vi "Teleop.vi"(0 "Call Context":T10) -> (6 "SubState 3":T2, 8 "SubState 4":T2, 9 "SubState 5":T9, 10 "Loop 4 Data":T1, 11 "Loop 3 Data":T5, 14 "SubState 0":T2=enum."driver control", 15 "Loop 1 Data":T7, 16 "Loop 0 Data":T8, 17 "SubState 1":T2, 18 "Loop 2 Data":T6, 19 "SubState 2":T2)   [LabVIEW 2013]
uses:
  typedefs/state machine/subStates.ctl
  <vilib>/Rock Robotics/WPI/DriverStation/WPI_DriverStationDerivedRobotMode.ctl
  typedefs/state machine/singleUseSubstate.ctl
  typedefs/loop datatypes/Loop 0 Datatype.ctl
  typedefs/loop datatypes/Loop 1 Datatype.ctl
  typedefs/loop datatypes/Loop 2 Datatype.ctl
  typedefs/loop datatypes/Loop 3 Datatype.ctl
  <vilib>/Rock Robotics/WPI/Joystick/WPI_JoystickDevRef.ctl
  <vilib>/Rock Robotics/WPI/Joystick/WPI_JoystickDeviceEnum.ctl
  typedefs/loop datatypes/Loop 4 Datatype.ctl
  typedefs/fg_getset.ctl
  typedefs/vision/vision enable.ctl
  <vilib>/Rock Robotics/WPI/Joystick/WPI_JoystickGetSetRefNum.vi
panel:
  out "Drive to DC":bool
  out "JS3":T3
  out "JS1":T3
  out "JS2":T3
  out "Exit Value":i32=-1
  # "Teleoperated Loop Data and Substates"
  # "Drive Loop"
  # "Loop 1"
  # "Loop 2"
  # "Loop 3"
  # "Loop 4"
  # "Pneumatics Loop"
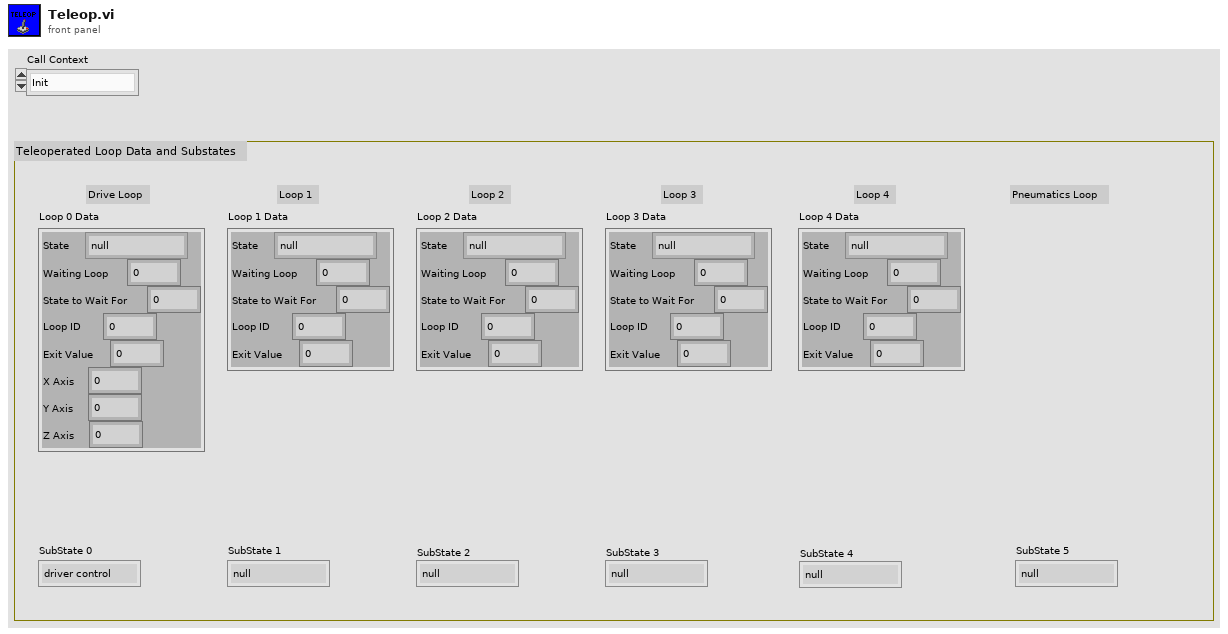
[diagram p1: front panel]
types:
  T1 = typedef "Loop 4 Datatype.ctl" = cluster{"State":T2, "Waiting Loop":i32, "State to Wait For":i32, "Loop ID":i32, "Exit Value":i32}
  T2 = typedef "subStates.ctl" = enum16{"null", "wait", "driver control", "auto", "manual override", "hold position", "rotate", "test", "end"}
  T3 = typedef "WPI_JoystickDevRef.ctl" = cluster{"Device":T4}
  T4 = typedef "WPI_JoystickDeviceEnum.ctl" = enum16{"USB 1", "USB 2", "USB 3", "USB 4", "Kinect 1", "Kinect 2"}
  T5 = typedef "Loop 3 Datatype.ctl" = cluster{"State":T2, "Waiting Loop":i32, "State to Wait For":i32, "Loop ID":i32, "Exit Value":i32}
  T6 = typedef "Loop 2 Datatype.ctl" = cluster{"State":T2, "Waiting Loop":i32, "State to Wait For":i32, "Loop ID":i32, "Exit Value":i32}
  T7 = typedef "Loop 1 Datatype.ctl" = cluster{"State":T2, "Waiting Loop":i32, "State to Wait For":i32, "Loop ID":i32, "Exit Value":i32}
  T8 = typedef "Loop 0 Datatype.ctl" = cluster{"State":T2, "Waiting Loop":i32, "State to Wait For":i32, "Loop ID":i32, "Exit Value":i32, "X Axis":dbl, "Y Axis":dbl, "Z Axis":dbl}
  T9 = typedef "singleUseSubstate.ctl" = enum16{"null", "wait", "shift high", "shift low", "end"}
  T10 = typedef "WPI_DriverStationDerivedRobotMode.ctl" = enum16{"Init", "Execute", "Stop"}
  T11 = cluster{"axis 1 (x)":dbl, "axis 2 (y)":dbl, "axis 3 (throttle)":dbl, "axis 4":dbl, "axis 5":dbl, "axis 6":dbl}
  T12 = typedef "vision enable.ctl" = enum16{"Enable", "Disable", "Stop"}
  T13 = typedef "fg_getset.ctl" = enum16{"Get", "Set"}
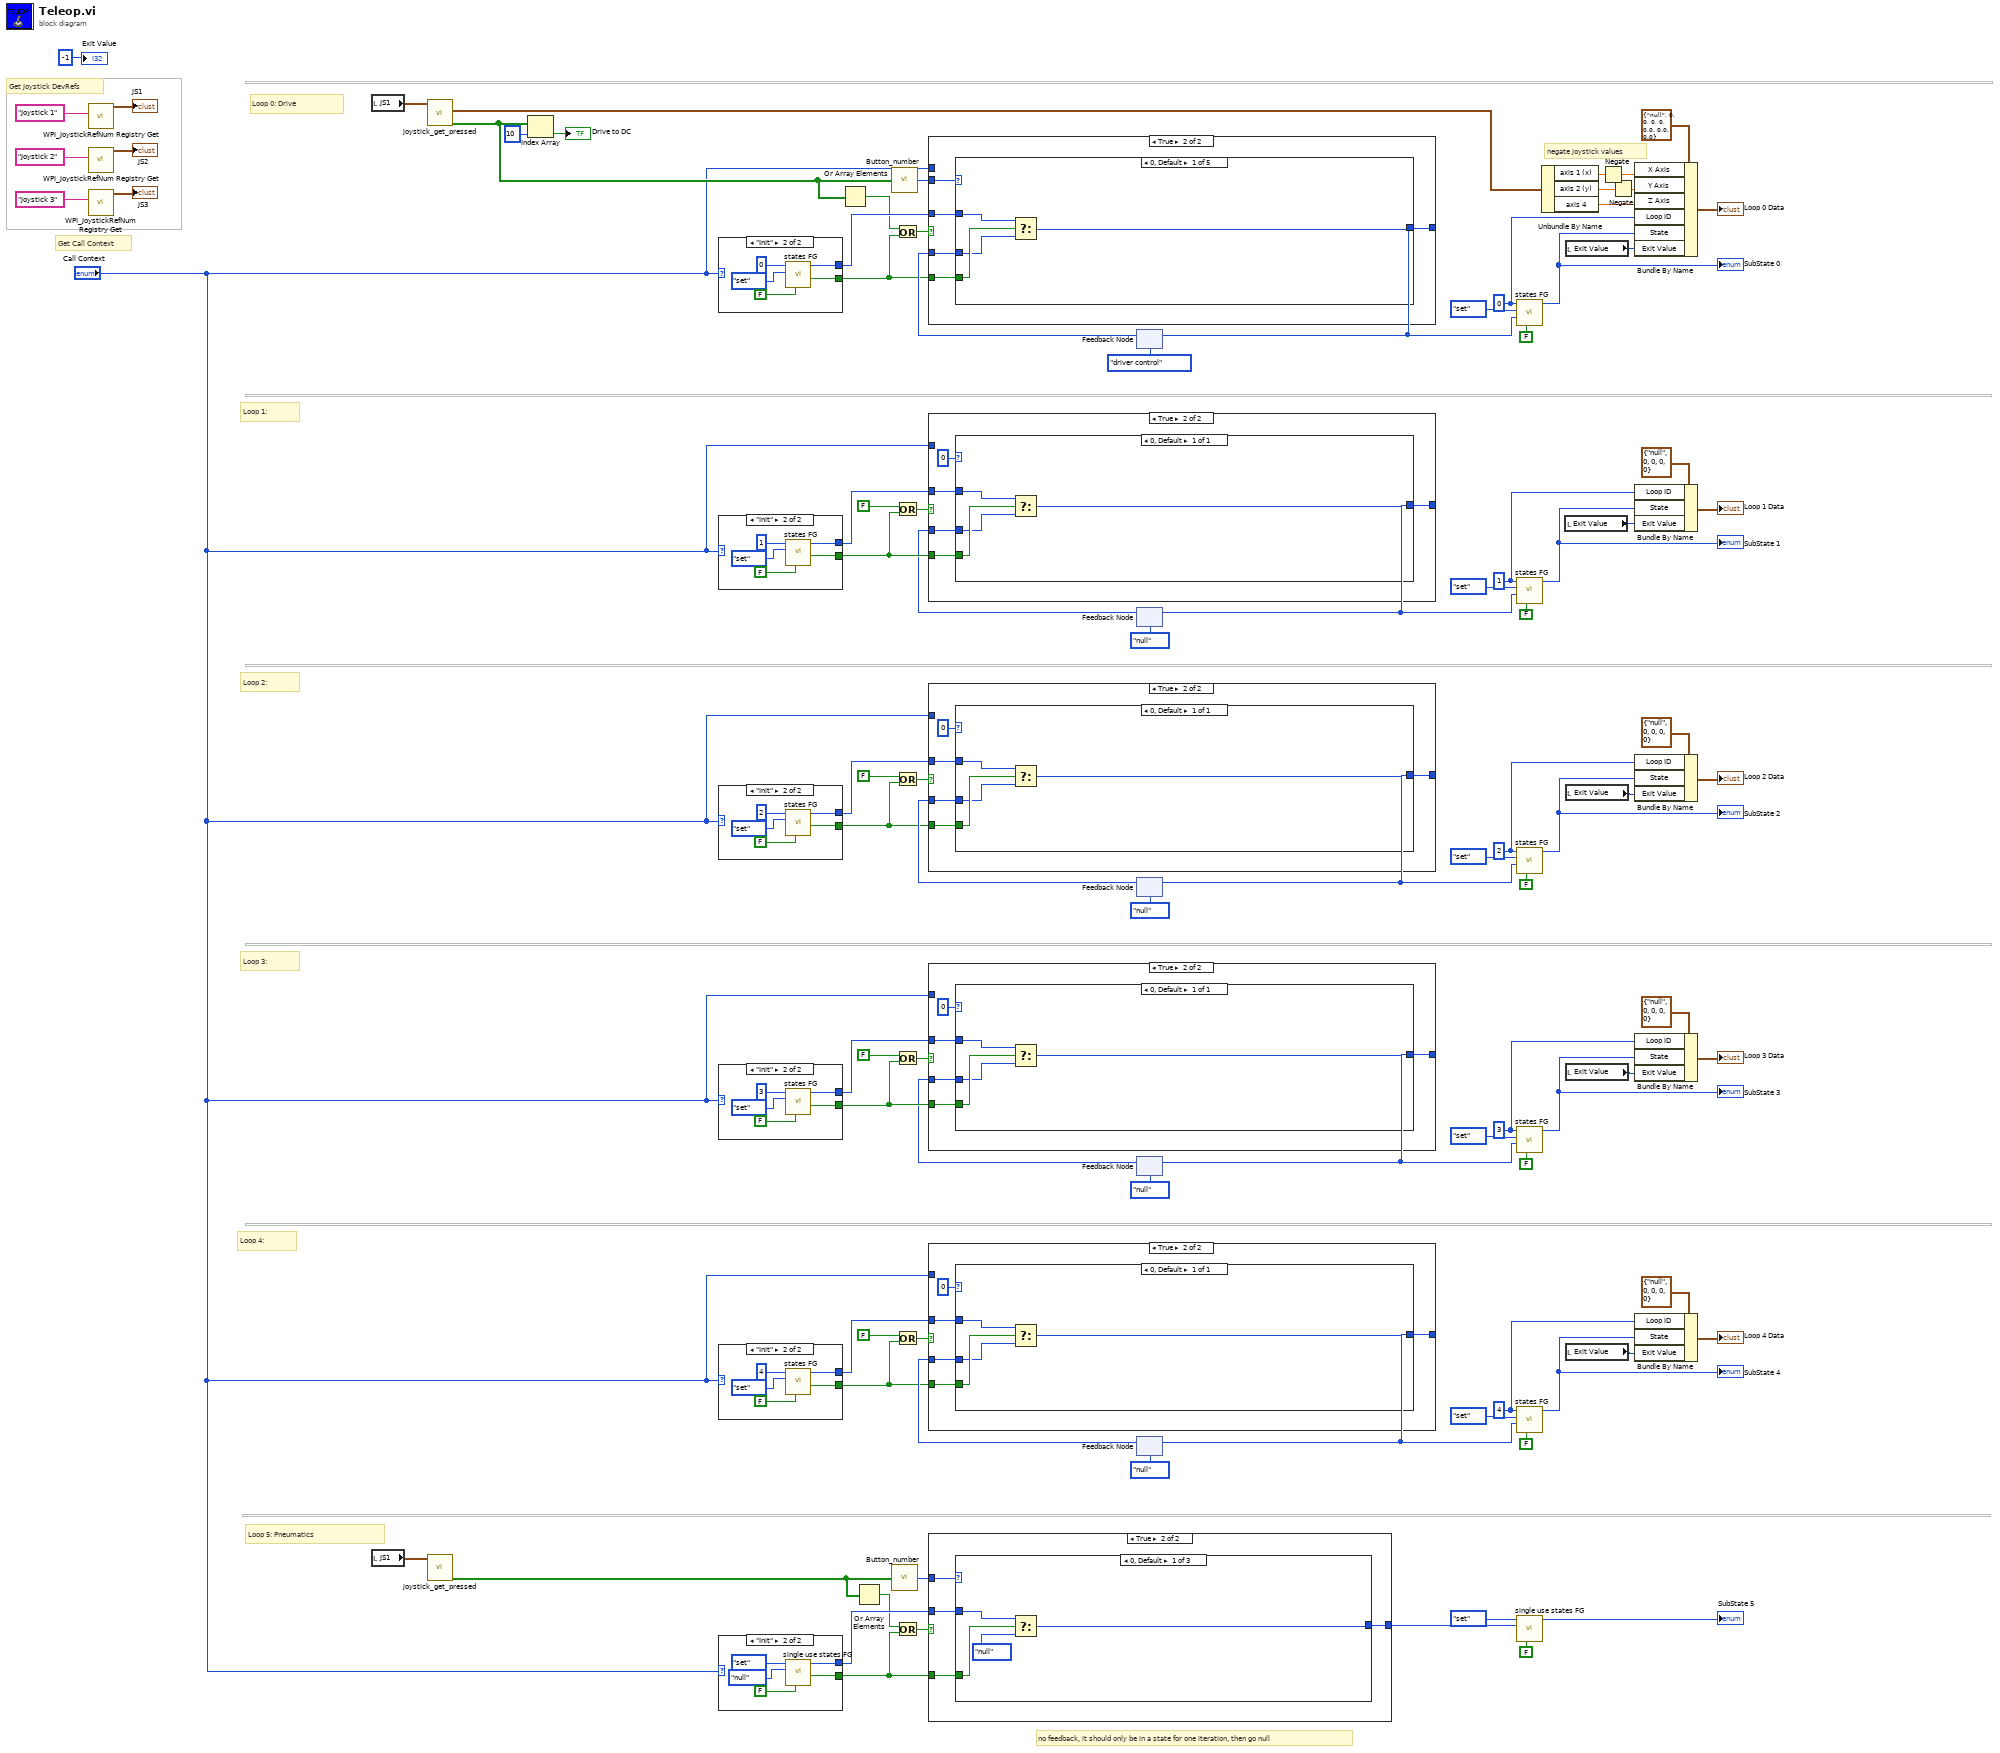
[diagram p0: block diagram]
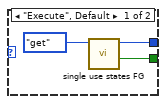
[diagram p2: hidden frame]
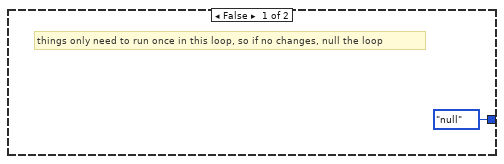
[diagram p3: hidden frame]
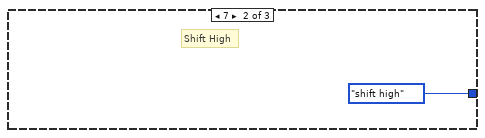
[diagram p4: hidden frame]
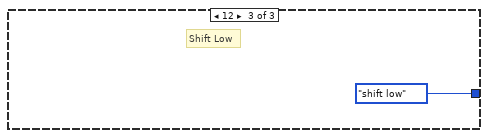
[diagram p5: hidden frame]
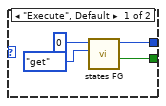
[diagram p6: hidden frame]
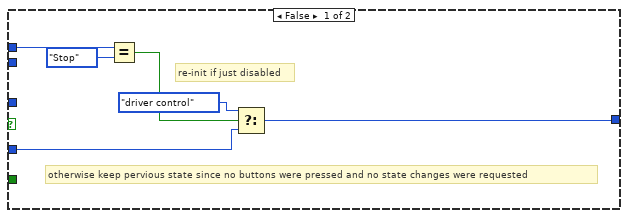
[diagram p7: hidden frame]
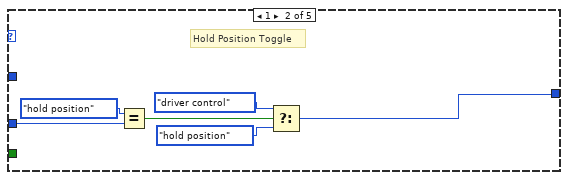
[diagram p8: hidden frame]
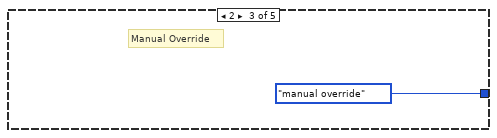
[diagram p9: hidden frame]
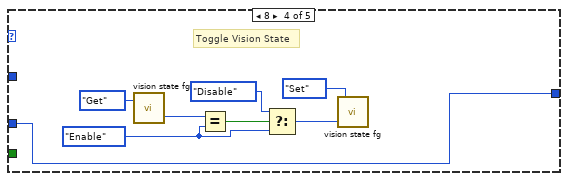
[diagram p10: hidden frame]
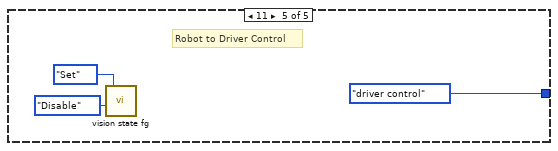
[diagram p11: hidden frame]
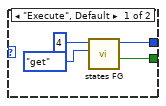
[diagram p12: hidden frame]
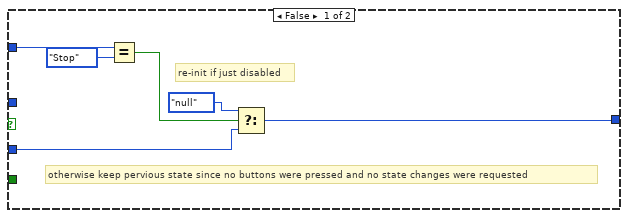
[diagram p13: hidden frame]
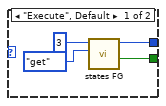
[diagram p14: hidden frame]
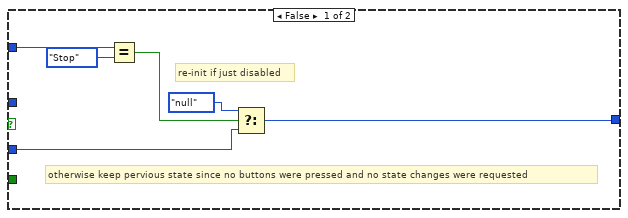
[diagram p15: hidden frame]
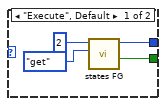
[diagram p16: hidden frame]
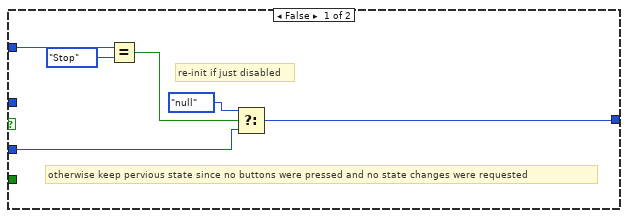
[diagram p17: hidden frame]
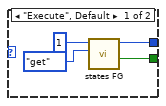
[diagram p18: hidden frame]
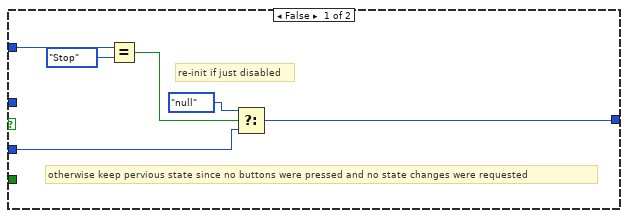
[diagram p19: hidden frame]
diagram:
  w39 = 0 ("Loop ID")
  w50 = 4 ("Loop ID")
  w65 = 3 ("Loop ID")
  w76 = 2 ("Loop ID")
  w94 = 1 ("Loop ID")
  # "no feedback, it should only be in a state for one iteration, then go null"
  # "negate joystick values"
  # "Loop 3:"
  # "Loop 2:"
  # "Loop 4:"
  # "Get Call Context"
  # "Get Joystick DevRefs"
  # "Loop 5: Pneumatics"
  # "Loop 1:"
  # "Loop 0: Drive"
  n1 = call <vilib>:"WPI_JoystickRefNum Registry Get.vi"("refnum name"="Joystick 1") -> ("JoystickDevRef"=→"JS1":T3)  [unwired: 9 in, 1 out]
  n2 = call <vilib>:"WPI_JoystickRefNum Registry Get.vi"("refnum name"="Joystick 2") -> ("JoystickDevRef"=→"JS2":T3)  [unwired: 9 in, 1 out]
  n3 = call <vilib>:"WPI_JoystickRefNum Registry Get.vi"("refnum name"="Joystick 3") -> ("JoystickDevRef"=→"JS3":T3)  [unwired: 9 in, 1 out]
  n4 = local read "JS1"() -> (w30:T3)
  n5 = local read "JS1"() -> (w12:T3)
  n6 = call "joystick_get_pressed.vi"("JoystickDevRef"=w30) -> ("Buttons Pressed?"=w20:bool[], "Axes"=w27:T11)  [unwired: 3 in, 2 out]
  n7 = call "joystick_get_pressed.vi"("JoystickDevRef"=w12) -> ("Buttons Pressed?"=w10:bool[])  [unwired: 3 in, 3 out]
  n8 = Index Array(array=w20, index=10) -> (element=→"Drive to DC":bool)
  n9 = case shown="\"Init\"" "Call Context" {
    tunnel: [w102 w107] -> w34
    tunnel: [w101 w105] -> w38
    frame "Execute", Default {
      n10 = call "states FG.vi"("menu (get)"=enum16{"set", "get"}."get", "Loop ID"=0) -> ("exit out"=w102:bool, "subState out"=w101:T2)  [unwired: 6 in, 2 out]
    }
    frame "Init" {
      n11 = call "states FG.vi"("exit in"=FALSE, "menu (get)"=enum16{"set", "get"}."set", "Loop ID"=0) -> ("exit out"=w107:bool, "subState out"=w105:T2)  [unwired: 5 in, 2 out]
    }
  }
  n12 = case shown="\"Init\"" "Call Context" {
    tunnel: [w111 w116] -> w100
    tunnel: [w110 w114] -> w96
    frame "Execute", Default {
      n13 = call "states FG.vi"("menu (get)"=enum16{"set", "get"}."get", "Loop ID"=1) -> ("exit out"=w111:bool, "subState out"=w110:T2)  [unwired: 6 in, 2 out]
    }
    frame "Init" {
      n14 = call "states FG.vi"("exit in"=FALSE, "menu (get)"=enum16{"set", "get"}."set", "Loop ID"=1) -> ("exit out"=w116:bool, "subState out"=w114:T2)  [unwired: 5 in, 2 out]
    }
  }
  n15 = case shown="\"Init\"" "Call Context" {
    tunnel: [w120 w125] -> w71
    tunnel: [w119 w123] -> w75
    frame "Execute", Default {
      n16 = call "states FG.vi"("menu (get)"=enum16{"set", "get"}."get", "Loop ID"=2) -> ("exit out"=w120:bool, "subState out"=w119:T2)  [unwired: 6 in, 2 out]
    }
    frame "Init" {
      n17 = call "states FG.vi"("exit in"=FALSE, "menu (get)"=enum16{"set", "get"}."set", "Loop ID"=2) -> ("exit out"=w125:bool, "subState out"=w123:T2)  [unwired: 5 in, 2 out]
    }
  }
  n18 = case shown="\"Init\"" "Call Context" {
    tunnel: [w129 w134] -> w70
    tunnel: [w128 w132] -> w66
    frame "Execute", Default {
      n19 = call "states FG.vi"("menu (get)"=enum16{"set", "get"}."get", "Loop ID"=3) -> ("exit out"=w129:bool, "subState out"=w128:T2)  [unwired: 6 in, 2 out]
    }
    frame "Init" {
      n20 = call "states FG.vi"("exit in"=FALSE, "menu (get)"=enum16{"set", "get"}."set", "Loop ID"=3) -> ("exit out"=w134:bool, "subState out"=w132:T2)  [unwired: 5 in, 2 out]
    }
  }
  n21 = case shown="\"Init\"" "Call Context" {
    tunnel: [w138 w143] -> w45
    tunnel: [w137 w141] -> w49
    frame "Execute", Default {
      n22 = call "states FG.vi"("menu (get)"=enum16{"set", "get"}."get", "Loop ID"=4) -> ("exit out"=w138:bool, "subState out"=w137:T2)  [unwired: 6 in, 2 out]
    }
    frame "Init" {
      n23 = call "states FG.vi"("exit in"=FALSE, "menu (get)"=enum16{"set", "get"}."set", "Loop ID"=4) -> ("exit out"=w143:bool, "subState out"=w141:T2)  [unwired: 5 in, 2 out]
    }
  }
  n24 = case shown="\"Init\"" "Call Context" {
    tunnel: [w148 w152] -> w16
    tunnel: [w147 w153] -> w15
    frame "Execute", Default {
      n25 = call "single use states FG.vi"("menu (get)"=enum16{"set", "get"}."get") -> ("exit out"=w148:bool, "substate out"=w147:T9)  [unwired: 7 in, 2 out]
    }
    frame "Init" {
      n26 = call "single use states FG.vi"("exit in"=FALSE, "substate"=singleUseSubstate."null", "menu (get)"=enum16{"set", "get"}."set") -> ("exit out"=w152:bool, "substate out"=w153:T9)  [unwired: 5 in, 2 out]
    }
  }
  n27 = Or Array Elements(Boolean array=w20) -> (logical OR=w19:bool)
  n28 = Or Array Elements(Boolean array=w10) -> (logical OR=w11:bool)
  n29 = call "Button_number.vi"("Button Array"=w20) -> ("Button Pressed"=w21:i32)
  n30 = call "Button_number.vi"("Button Array"=w10) -> ("Button Pressed"=w9:i32)
  n31 = Or(x=w19, y=w34) -> (x .or. y?=w42:bool)
  n32 = Or(x=FALSE, y=w100) -> (x .or. y?=w83:bool)
  n33 = Or(x=FALSE, y=w71) -> (x .or. y?=w79:bool)
  n34 = Or(x=FALSE, y=w70) -> (x .or. y?=w62:bool)
  n35 = Or(x=FALSE, y=w45) -> (x .or. y?=w53:bool)
  n36 = Or(x=w11, y=w16) -> (x .or. y?=w14:bool)
  n37 = case shown="True" w14 {
    tunnel: [singleUseSubstate."null" ("substate out") w157] -> w8
    tunnel: w15 -> [_ w158]
    tunnel: w16 -> [_ w156]
    tunnel: w9 -> [_ w155]
    frame False {
      # "things only need to run once in this loop, so if no changes, null the loop"
    }
    frame True {
      n38 = case shown="0, Default" w155 {
        tunnel: w158 -> [w161 _ _]
        tunnel: [w160 singleUseSubstate."shift high" ("f") singleUseSubstate."shift low" ("f")] -> w157
        tunnel: w156 -> [w162 _ _]
        frame 0, Default {
          n39 = Select(t=w161, s=w162, f=singleUseSubstate."null") -> (s? t:f=w160:T9)
        }
        frame 7 {
          # "Shift High"
        }
        frame 12 {
          # "Shift Low"
        }
      }
    }
  }
  n40 = feedback #1(subStates."driver control" ("Drive SubState")) -> (w41:T2)
  n41 = case shown="True" w42 {
    tunnel: w41 -> [w167 w174]
    tunnel: [w165 w173] -> w33
    tunnel: w38 -> [_ w175]
    tunnel: w34 -> [_ w172]
    tunnel: "Call Context" -> [w170 _]
    tunnel: w21 -> [_ w171]
    frame False {
      # "re-init if just disabled"
      # "otherwise keep pervious state since no buttons were pressed and no state changes were requested"
      n42 = Equal?(x=w170, y=WPI_DriverStationDerivedRobotMode."Stop") -> (x = y?=w168:bool)
      n43 = Select(t=subStates."driver control", s=w168, f=w167) -> (s? t:f=w165:T2)
    }
    frame True {
      n44 = case shown="0, Default" w171 {
        tunnel: w175 -> [w178 _ _ _ _]
        tunnel: w174 -> [w177 w185 _ w187 _]
        tunnel: [w176 w180 subStates."manual override" ("Drive SubState") w187 subStates."driver control" ("Drive SubState")] -> w173
        tunnel: w172 -> [w179 _ _ _ _]
        frame 0, Default {
          n45 = Select(t=w178, s=w179, f=w177) -> (s? t:f=w176:T2)
        }
        frame 1 {
          # "Hold Position Toggle"
          n46 = Equal?(x=subStates."hold position", y=w185) -> (x = y?=w183:bool)
          n47 = Select(t=subStates."driver control" ("Drive SubState"), s=w183, f=subStates."hold position" ("Drive SubState")) -> (s? t:f=w180:T2)
        }
        frame 2 {
          # "Manual Override"
        }
        frame 8 {
          w192 = vision_enable."Enable" ("y")
          # "Toggle Vision State"
          n48 = call "vision state fg.vi"("Menu"=fg_getset."Get") -> ("State Out"=w190:T12)  [unwired: 1 in, 1 out]
          n49 = Equal?(x=w190, y=w192) -> (x = y?=w191:bool)
          n50 = Select(t=vision_enable."Disable" ("y"), s=w191, f=w192) -> (s? t:f=w194:T12)
          n51 = call "vision state fg.vi"("Action"=w194, "Menu"=fg_getset."Set") -> ()  [unwired: 2 out]
        }
        frame 11 {
          # "Robot to Driver Control"
          n52 = call "vision state fg.vi"("Action"=vision_enable."Disable", "Menu"=fg_getset."Set") -> ()  [unwired: 2 out]
        }
      }
    }
  }
  n53 = feedback-in #1(w33) -> ()
  n54 = feedback #2(subStates."null" ("Drive SubState")) -> (w84:T2)
  n55 = case shown="True" w83 {
    tunnel: w84 -> [w200 w207]
    tunnel: [w198 w206] -> w81
    tunnel: w96 -> [_ w208]
    tunnel: w100 -> [_ w205]
    tunnel: "Call Context" -> [w203 _]
    frame False {
      # "re-init if just disabled"
      # "otherwise keep pervious state since no buttons were pressed and no state changes were requested"
      n56 = Equal?(x=w203, y=WPI_DriverStationDerivedRobotMode."Stop") -> (x = y?=w201:bool)
      n57 = Select(t=subStates."null", s=w201, f=w200) -> (s? t:f=w198:T2)
    }
    frame True {
      n58 = case shown="0, Default" 0 ("Button Pressed") {
        tunnel: w208 -> [w211]
        tunnel: w207 -> [w210]
        tunnel: [w209] -> w206
        tunnel: w205 -> [w212]
        frame 0, Default {
          n59 = Select(t=w211, s=w212, f=w210) -> (s? t:f=w209:T2)
        }
      }
    }
  }
  n60 = feedback-in #2(w81) -> ()
  n61 = feedback #3(subStates."null" ("Drive SubState")) -> (w78:T2)
  n62 = case shown="True" w79 {
    tunnel: w78 -> [w215 w222]
    tunnel: [w213 w221] -> w60
    tunnel: w75 -> [_ w223]
    tunnel: w71 -> [_ w220]
    tunnel: "Call Context" -> [w218 _]
    frame False {
      # "re-init if just disabled"
      # "otherwise keep pervious state since no buttons were pressed and no state changes were requested"
      n63 = Equal?(x=w218, y=WPI_DriverStationDerivedRobotMode."Stop") -> (x = y?=w216:bool)
      n64 = Select(t=subStates."null", s=w216, f=w215) -> (s? t:f=w213:T2)
    }
    frame True {
      n65 = case shown="0, Default" 0 ("Button Pressed") {
        tunnel: w223 -> [w226]
        tunnel: w222 -> [w225]
        tunnel: [w224] -> w221
        tunnel: w220 -> [w227]
        frame 0, Default {
          n66 = Select(t=w226, s=w227, f=w225) -> (s? t:f=w224:T2)
        }
      }
    }
  }
  n67 = feedback-in #3(w60) -> ()
  n68 = feedback #4(subStates."null" ("Drive SubState")) -> (w63:T2)
  n69 = case shown="True" w62 {
    tunnel: w63 -> [w230 w237]
    tunnel: [w228 w236] -> w55
    tunnel: w66 -> [_ w238]
    tunnel: w70 -> [_ w235]
    tunnel: "Call Context" -> [w233 _]
    frame False {
      # "re-init if just disabled"
      # "otherwise keep pervious state since no buttons were pressed and no state changes were requested"
      n70 = Equal?(x=w233, y=WPI_DriverStationDerivedRobotMode."Stop") -> (x = y?=w231:bool)
      n71 = Select(t=subStates."null", s=w231, f=w230) -> (s? t:f=w228:T2)
    }
    frame True {
      n72 = case shown="0, Default" 0 ("Button Pressed") {
        tunnel: w238 -> [w241]
        tunnel: w237 -> [w240]
        tunnel: [w239] -> w236
        tunnel: w235 -> [w242]
        frame 0, Default {
          n73 = Select(t=w241, s=w242, f=w240) -> (s? t:f=w239:T2)
        }
      }
    }
  }
  n74 = feedback-in #4(w55) -> ()
  n75 = feedback #5(subStates."null" ("Drive SubState")) -> (w52:T2)
  n76 = case shown="True" w53 {
    tunnel: w52 -> [w245 w252]
    tunnel: [w243 w251] -> w44
    tunnel: w49 -> [_ w253]
    tunnel: w45 -> [_ w250]
    tunnel: "Call Context" -> [w248 _]
    frame False {
      # "re-init if just disabled"
      # "otherwise keep pervious state since no buttons were pressed and no state changes were requested"
      n77 = Equal?(x=w248, y=WPI_DriverStationDerivedRobotMode."Stop") -> (x = y?=w246:bool)
      n78 = Select(t=subStates."null", s=w246, f=w245) -> (s? t:f=w243:T2)
    }
    frame True {
      n79 = case shown="0, Default" 0 ("Button Pressed") {
        tunnel: w253 -> [w256]
        tunnel: w252 -> [w255]
        tunnel: [w254] -> w251
        tunnel: w250 -> [w257]
        frame 0, Default {
          n80 = Select(t=w256, s=w257, f=w255) -> (s? t:f=w254:T2)
        }
      }
    }
  }
  n81 = feedback-in #5(w44) -> ()
  n82 = call "states FG.vi"("exit in"=FALSE, "subState in"=w33, "menu (get)"=enum16{"set", "get"}."set", "Loop ID"=w39) -> ("subState out"=w2:T2)  [unwired: 4 in, 3 out]
  "SubState 0" <- w2
  n83 = call "states FG.vi"("exit in"=FALSE, "subState in"=w81, "menu (get)"=enum16{"set", "get"}."set", "Loop ID"=w94) -> ("subState out"=w3:T2)  [unwired: 4 in, 3 out]
  "SubState 1" <- w3
  n84 = call "states FG.vi"("exit in"=FALSE, "subState in"=w60, "menu (get)"=enum16{"set", "get"}."set", "Loop ID"=w76) -> ("subState out"=w4:T2)  [unwired: 4 in, 3 out]
  "SubState 2" <- w4
  n85 = call "states FG.vi"("exit in"=FALSE, "subState in"=w55, "menu (get)"=enum16{"set", "get"}."set", "Loop ID"=w65) -> ("subState out"=w5:T2)  [unwired: 4 in, 3 out]
  "SubState 3" <- w5
  n86 = call "states FG.vi"("exit in"=FALSE, "subState in"=w44, "menu (get)"=enum16{"set", "get"}."set", "Loop ID"=w50) -> ("subState out"=w6:T2)  [unwired: 4 in, 3 out]
  "SubState 4" <- w6
  n87 = call "single use states FG.vi"("exit in"=FALSE, "substate"=w8, "menu (get)"=enum16{"set", "get"}."set") -> ("substate out"=→"SubState 5":T9)  [unwired: 5 in, 3 out]
  n88 = Unbundle By Name(w27) -> ("axis 1 (x)"=w26:dbl, "axis 2 (y)"=w25:dbl, "axis 4"=w24:dbl)
  n89 = local read "Exit Value"() -> (w92:i32)
  n90 = local read "Exit Value"() -> (w40:i32)
  n91 = local read "Exit Value"() -> (w77:i32)
  n92 = local read "Exit Value"() -> (w64:i32)
  n93 = local read "Exit Value"() -> (w51:i32)
  n94 = Negate(x=w26) -> (-x=w23:dbl)
  n95 = Negate(x=w25) -> (-x=w22:dbl)
  n96 = Bundle By Name(cluster=T8 {"State"=enum."null", "Waiting Loop"=0, "State to Wait For"=0, "Loop ID"=0, "Exit Value"=0, "X Axis"=0.0, "Y Axis"=0.0, "Z Axis"=0.0} ("Cluster"), "X Axis"=w23, "Y Axis"=w22, "Z Axis"=w24, "Loop ID"=w39, "State"=w2, "Exit Value"=w40) -> (→"Loop 0 Data":T8)
  n97 = Bundle By Name(cluster=T7 {"State"=enum."null", "Waiting Loop"=0, "State to Wait For"=0, "Loop ID"=0, "Exit Value"=0} ("Cluster"), "Loop ID"=w94, "State"=w3, "Exit Value"=w92) -> (→"Loop 1 Data":T7)
  n98 = Bundle By Name(cluster=T6 {"State"=enum."null", "Waiting Loop"=0, "State to Wait For"=0, "Loop ID"=0, "Exit Value"=0} ("Loop 2 Data"), "Loop ID"=w76, "State"=w4, "Exit Value"=w77) -> (→"Loop 2 Data":T6)
  n99 = Bundle By Name(cluster=T5 {"State"=enum."null", "Waiting Loop"=0, "State to Wait For"=0, "Loop ID"=0, "Exit Value"=0} ("Loop 3 Data"), "Loop ID"=w65, "State"=w5, "Exit Value"=w64) -> (→"Loop 3 Data":T5)
  n100 = Bundle By Name(cluster=T1 {"State"=enum."null", "Waiting Loop"=0, "State to Wait For"=0, "Loop ID"=0, "Exit Value"=0} ("Loop 4 Data"), "Loop ID"=w50, "State"=w6, "Exit Value"=w51) -> (→"Loop 4 Data":T1)
  "Exit Value" <- -1 ("Exit Value")
